vi "Get Dependencies.vi"(8 "error in (no error)":errorcluster, 11 "Instrument in":refnum<class "Instrument.lvclass">) -> (0 "error out":errorcluster, 2 "Dependencies":T1, 3 "Instrument out":refnum<class "Instrument.lvclass">)   [LabVIEW 2019, in "Instrument.lvclass"]
uses:
  Instrument.lvclass
  Logger.PGSQL/Logger.PGSQL.lvclass
  Typedefs/Dependencies--Cluster.ctl
  <userlib>/LevyLab/RemoteControl/RemoteControl.lvclass
  Logger.Error/Logger.Error.lvclass
  <userlib>/LevyLab/Configuration/Configuration.lvclass
  C:/Program Files (x86)/National Instruments/LabVIEW 2019/vi.lib/JKI/JKI SMO/SMO/SMO.lvclass
  Instrument.lvclass/Instrument.ctl
  <vilib>/JKI/JKI SMO/SMO/SMO.lvclass
  <vilib>/regexp/Match Regular Expression.xnode
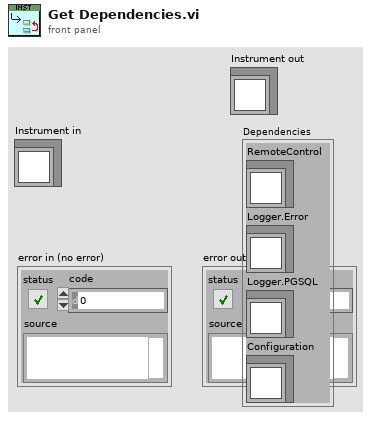
[diagram p1: front panel]
types:
  T1 = typedef "Instrument.lvclass/Dependencies--Cluster.ctl" = cluster{"RemoteControl":refnum<class "RemoteControl.lvclass">, "Logger.Error":refnum<class "Logger.Error.lvclass">, "Logger.PGSQL":refnum<class "Logger.PGSQL.lvclass">, "Configuration":refnum<class "Configuration.lvclass">}
  T2 = cluster{"RemoteControl":refnum<class "RemoteControl.lvclass">, "Logger.Error":refnum<class "Logger.Error.lvclass">, "Logger.PGSQL":refnum<class "Logger.PGSQL.lvclass">, "Configuration":refnum<class "Configuration.lvclass">}
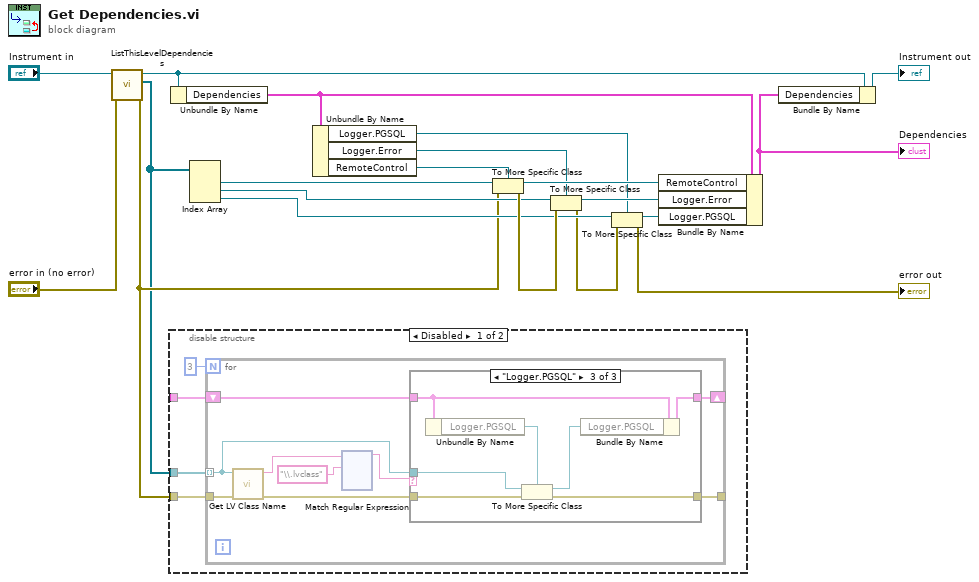
[diagram p0: block diagram]
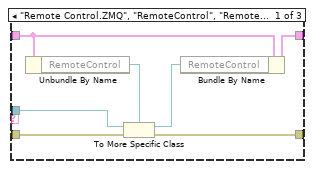
[diagram p2: hidden frame]
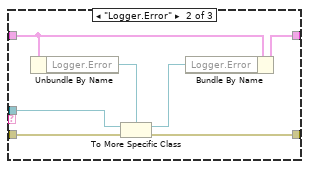
[diagram p3: hidden frame]
diagram:
  n1 = call <vilib>:"ListThisLevelDependencies.vi"("error in (no error)"="error in (no error)", "SMO in"="Instrument in") -> ("error out"=w11:errorcluster, "[My Dependencies]"=w2:refnum<class "SMO.lvclass">[], "SMO out"=w9:refnum<class "Instrument.lvclass">)  [unwired: 7 in]
  n2 = disable-structure shown="Disabled" {
    disable-tunnel: w2 -> [w24 _]
    disable-tunnel: _ -> [w23 _]
    disable-tunnel: w11 -> [w22 _]
    frame Disabled {
      n3 = for {
        N: 3 -> [_]
        tunnel: w22 -> [w30]
        tunnel: [w32] -> _
        shift-right: [w31] -> _
        shift-left: w23 -> [w33]
        tunnel: w24 -> [w27] mode=indexing
        n4 = call <vilib>:"Get LV Class Name.vi"("error in (no error)"=w30, "object"=w27) -> ("error out"=w29:errorcluster, "class name"=w28:string)  [unwired: 8 in]
        n5 = xnode "Match Regular Expression"("input string"=w28, "regular expression"="\\.lvclass") -> ("before match"=w26:string)  [unwired: 4 in, 4 out]
        n6 = case shown="\"Logger.PGSQL\"" w26 {
          tunnel: w33 -> [w154 w161 w168]
          tunnel: [w152 w159 w166] -> w32
          tunnel: [w151 w158 w165] -> w31
          tunnel: w27 -> [w150 w157 w164]
          tunnel: w29 -> [w148 w155 w162]
          frame "Remote Control.ZMQ", "RemoteControl", "RemoteControl.STM", Default {
            n7 = Unbundle By Name(w154) -> ("RemoteControl"=w153:refnum<class "RemoteControl.lvclass">)
            n8 = To More Specific Class(target class=w153, reference=w150, error in=w148) -> (specific class reference=w149:refnum<class "RemoteControl.lvclass">, error out=w152:errorcluster)
            n9 = Bundle By Name(cluster=w154, "RemoteControl"=w149) -> (w151:T2)
          }
          frame "Logger.Error" {
            n10 = Unbundle By Name(w161) -> ("Logger.Error"=w160:refnum<class "Logger.Error.lvclass">)
            n11 = To More Specific Class(target class=w160, reference=w157, error in=w155) -> (specific class reference=w156:refnum<class "Logger.Error.lvclass">, error out=w159:errorcluster)
            n12 = Bundle By Name(cluster=w161, "Logger.Error"=w156) -> (w158:T2)
          }
          frame "Logger.PGSQL" {
            n13 = Unbundle By Name(w168) -> ("Logger.PGSQL"=w167:refnum<class "Logger.PGSQL.lvclass">)
            n14 = To More Specific Class(target class=w167, reference=w164, error in=w162) -> (specific class reference=w163:refnum<class "Logger.PGSQL.lvclass">, error out=w166:errorcluster)
            n15 = Bundle By Name(cluster=w168, "Logger.PGSQL"=w163) -> (w165:T2)
          }
        }
      }
    }
    frame Enabled {
    }
  }
  n16 = Unbundle By Name(w9) -> ("Dependencies"=w5:T2)
  n17 = Index Array(array=w2) -> (element #1=w20:refnum<class "SMO.lvclass">, element #2=w15:refnum<class "SMO.lvclass">, element #3=w14:refnum<class "SMO.lvclass">)  [unwired: 3 in]
  n18 = Unbundle By Name(w5) -> ("Logger.PGSQL"=w6:refnum<class "Logger.PGSQL.lvclass">, "Logger.Error"=w7:refnum<class "Logger.Error.lvclass">, "RemoteControl"=w8:refnum<class "RemoteControl.lvclass">)
  n19 = To More Specific Class(target class=w8, reference=w20, error in=w11) -> (specific class reference=w18:refnum<class "RemoteControl.lvclass">, error out=w16:errorcluster)
  n20 = To More Specific Class(target class=w7, reference=w15, error in=w16) -> (specific class reference=w13:refnum<class "Logger.Error.lvclass">, error out=w4:errorcluster)
  n21 = To More Specific Class(target class=w6, reference=w14, error in=w4) -> (specific class reference=w12:refnum<class "Logger.PGSQL.lvclass">, error out=→"error out":errorcluster)
  n22 = Bundle By Name(cluster=w5, "RemoteControl"=w18, "Logger.Error"=w13, "Logger.PGSQL"=w12) -> (w1:T2)
  "Dependencies" <- w1
  n23 = Bundle By Name(cluster=w9, "Dependencies"=w1) -> (→"Instrument out":refnum<class "Instrument.lvclass">)
